vi "Generate Unique Header.vi"(8 "error in":errorcluster, 11 "CRDS Data in":refnum<class "CRDS Data.lvclass">) -> (0 "error out":errorcluster, 2 "Header":string[](array[string]), 3 "CRDS Data out":refnum<class "CRDS Data.lvclass">)   [LabVIEW 2014, in "CRDS Lib.lvlib" / "CRDS Data.lvclass"]
uses:
  CRDS Data.lvclass
  CRDS Data.lvclass/CRDS Data.ctl
  Cell/CRDS Cell Data.lvclass
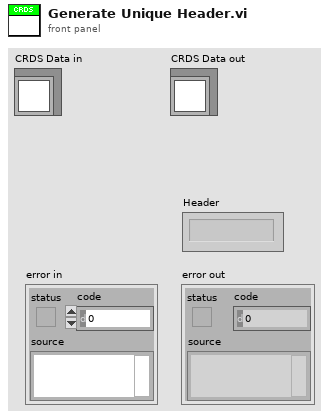
[diagram p1: front panel]
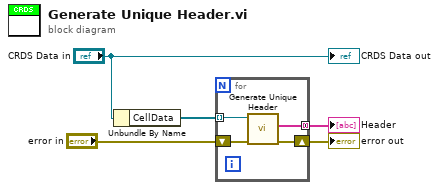
[diagram p0: block diagram]
diagram:
  n1 = Unbundle By Name("CRDS Data in") -> ("CellData"=w5:refnum<class "CRDS Cell Data.lvclass">[])
  n2 = for {
    tunnel: w5 -> [w9] mode=indexing
    tunnel: [w8] -> w4 mode=concatenating
    shift-right: [w6] -> w1
    shift-left: "error in" -> [w7]
    n3 = call-dynamic "Generate Unique Header.vi"("error in"=w7, "CRDS Cell Data in"=w9) -> ("error out"=w6:errorcluster, "Header"=w8:string[])  [unwired: 7 in, 1 out]
  }
  "error out" <- w1
  "Header" <- w4
  "CRDS Data out" <- "CRDS Data in"
